vi "Drive Curve.vi"(8 "Operator":dbl, 10 "Left":dbl, 11 "Right":dbl) -> (2 "Left":dbl, 3 "Right":dbl)   [LabVIEW 2016]
doc: "This VI curves the throttle of a tank drive using a user specified operator. Values between 1.5 and 3 are suggested.\n\nCreated by Team 4130 for use in the 2016-2017 FRC season"
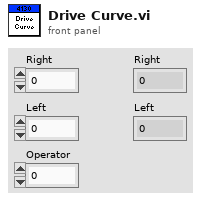
[diagram p1: front panel]
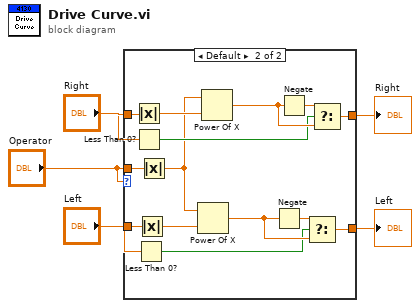
[diagram p0: block diagram]
diagram:
  n1 = case shown="Default" "Operator" {
    tunnel: [w7 w20] -> w5
    tunnel: [w6 w15] -> w4
    tunnel: "Left" -> [w6 w14]
    tunnel: "Right" -> [w7 w12]
    tunnel: "Operator" -> [_ w9]
    frame 0 {
    }
    frame Default {
      n2 = Absolute Value(x=w12) -> (abs(x)=w13:dbl)
      n3 = Less Than 0?(x=w12) -> (x < 0?=w11:bool)
      n4 = Less Than 0?(x=w14) -> (x < 0?=w10:bool)
      n5 = Absolute Value(x=w14) -> (abs(x)=w21:dbl)
      n6 = Absolute Value(x=w9) -> (abs(x)=w8:dbl)
      n7 = Power Of X(1:w21, 2:w8) -> (0:w16:dbl)
      n8 = Power Of X(1:w13, 2:w8) -> (0:w18:dbl)
      n9 = Negate(x=w16) -> (-x=w17:dbl)
      n10 = Negate(x=w18) -> (-x=w19:dbl)
      n11 = Select(t=w17, s=w10, f=w16) -> (s? t:f=w15:dbl)
      n12 = Select(t=w19, s=w11, f=w18) -> (s? t:f=w20:dbl)
    }
  }
  "Right" <- w5
  "Left" <- w4
